vi "Async Spawn Root.vi"(4 "UID":string, 6 "Core Actors":refnum<class "Actor.lvclass">[](array[class]), 9 "Mid Actors":refnum<class "Actor.lvclass">[](array[class]), 10 "Edge Actors":refnum<class "Actor.lvclass">[](array[class])) -> (0 "Error out":errorcluster, 2 "Root Attributes":refnum<class "Attributes.lvclass">)   [LabVIEW 2020, in "jettl.lvlib"]
uses:
  jettl.lvlib
  Actor/Actor.lvclass
  Attributes/Attributes.lvclass
  Transport/Transport.lvclass
  Msg/Msg.lvclass
  Base Attributes/Base Attributes.lvlib
  Msgs.ctl
  Attributes.ctl
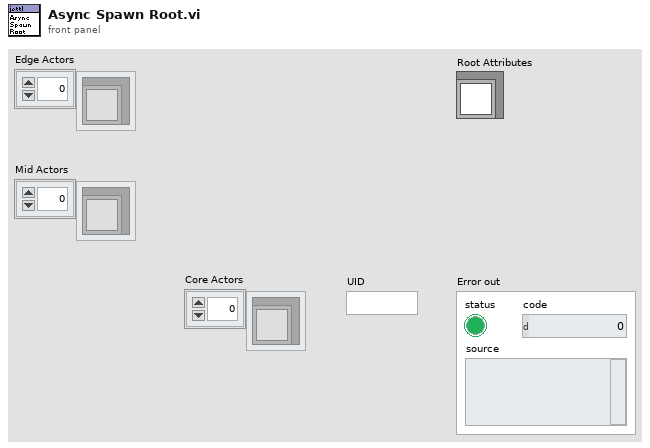
[diagram p1: front panel]
types:
  T1 = typedef "jettl.lvlib/Attributes.ctl" = cluster{"Unified Msgs":T2, "Edge Actors":refnum<class "Actor.lvclass">[], "Core Actors":refnum<class "Actor.lvclass">[], "Parent Attributes":refnum<class "Attributes.lvclass">, "Root":bool, "App Ref":refnum<vi>, "UID":string, "Transport":refnum<class "Transport.lvclass">, "VI Ref":refnum<vi>, "Actors":refnum<class "Actor.lvclass">[]}
  T2 = typedef "jettl.lvlib/Msgs.ctl" = set{refnum<class "Msg.lvclass">}
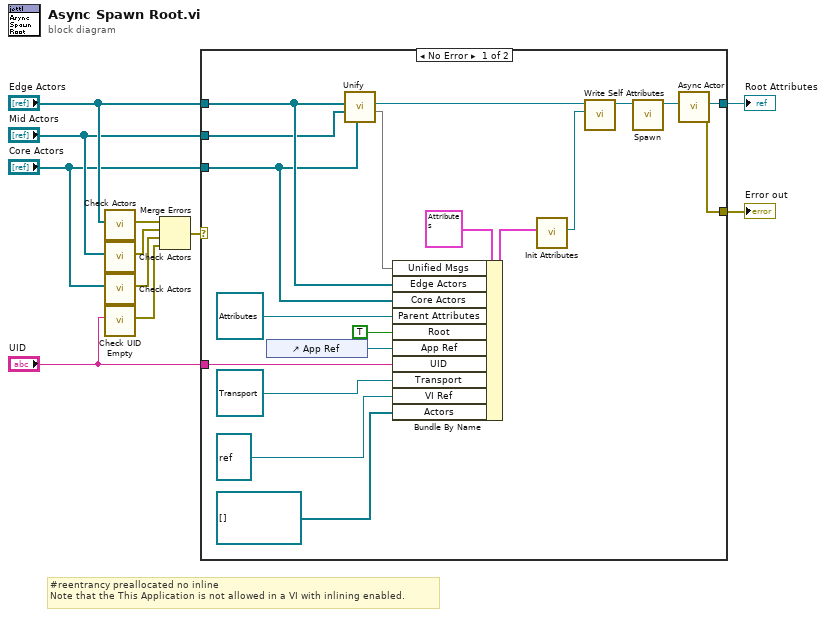
[diagram p0: block diagram]
diagram:
  # "#reentrancy preallocated no inline\nNote that the This Application is not allowed in a VI with inlining enabled."
  n1 = call "Check Actors.vi"("Actors"="Edge Actors") -> ("Error"=w1:errorcluster)  [unwired: 10 in]
  n2 = call "Check Actors.vi"("Actors"="Mid Actors") -> ("Error"=w8:errorcluster)  [unwired: 10 in]
  n3 = call "Check Actors.vi"("Actors"="Core Actors") -> ("Error"=w2:errorcluster)  [unwired: 10 in]
  n4 = call "Check UID Empty.vi"("UID"="UID") -> ("Error"=w7:errorcluster)  [unwired: 10 in]
  n5 = Merge Errors(w1, w8, w2, w7) -> (w9:errorcluster)
  n6 = case shown="No Error" w9 {
    selector: w9 -> [_ w31]
    tunnel: "Edge Actors" -> [w16 _]
    tunnel: [w30 w31] -> w11
    tunnel: [w29 _] -> w10
    tunnel: "UID" -> [w26 _]
    tunnel: "Mid Actors" -> [w15 _]
    tunnel: "Core Actors" -> [w14 _]
    frame No Error {
      n7 = control-ref of="App Ref"() -> (w27:refnum<vi>)
      n8 = call "Unify.vi"("Core Actors"=w14, "Mid Actors"=w15, "Edge Actors"=w16) -> ("Unified Msgs"=w12:T2, "Unified Actor"=w13:refnum<class "Actor.lvclass">)  [unwired: 7 in]
      n9 = Bundle By Name(cluster=T1 {"Unified Msgs"={}, "Edge Actors"=[], "Core Actors"=[], "Parent Attributes"=refnum, "Root"=FALSE, "App Ref"=refnum, "UID"="", "Transport"=refnum, "VI Ref"=refnum, "Actors"=[]} ("Attributes"), "Unified Msgs"=w12, "Edge Actors"=w16, "Core Actors"=w14, "Parent Attributes"=refnum<class "Attributes.lvclass"> refnum, "Root"=TRUE, "App Ref"=w27, "UID"=w26, "Transport"=refnum<class "Transport.lvclass"> refnum, "VI Ref"=refnum<vi> refnum ("Actor Ref"), "Actors"=refnum<class "Actor.lvclass">[] []) -> (w19:T1)
      n10 = call "Init Attributes.vi"("Attributes"=w19) -> ("Attributes"=w28:refnum<class "Attributes.lvclass">)  [unwired: 10 in]
      n11 = call-dynamic "Write Self Attributes.vi"("Self Attributes"=w28, "Actor in"=w13) -> ("Actor out"=w18:refnum<class "Actor.lvclass">)  [unwired: 9 in]
      n12 = call-dynamic "Spawn.vi"("Actor in"=w18) -> ("Actor out"=w17:refnum<class "Actor.lvclass">)  [unwired: 10 in]
      n13 = call "Async Actor.vi"("Unified Actor"=w17) -> ("Error out"=w30:errorcluster, "Child Attributes"=w29:refnum<class "Attributes.lvclass">)  [unwired: 9 in]
    }
    frame Error {
    }
  }
  "Error out" <- w11
  "Root Attributes" <- w10
